vi "Constant_Extension_TICArray.vi"() -> (0 "Information Array Name String":string="tic")   [LabVIEW 2018]
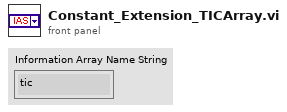
[diagram p1: front panel]
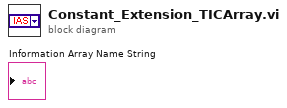
[diagram p0: block diagram]
diagram:
